vi "Serialize To Inputs.vi"(0 "Input 6":variant, 4 "Input 5":variant, 6 "Input 4":variant, 8 "Input 3":variant, 9 "Input 2":variant, 10 "Input 1":variant, 11 "Base Queue in":refnum<class "Base Queue.lvclass">) -> (3 "Base Queue out":refnum<class "Base Queue.lvclass">)   [LabVIEW 2021, in "jettl.lvlib" / "Base Queue.lvlib" / "Base Queue.lvclass"]
uses:
  Base Queue.lvclass
  Base Queue.lvclass/Base Queue.ctl
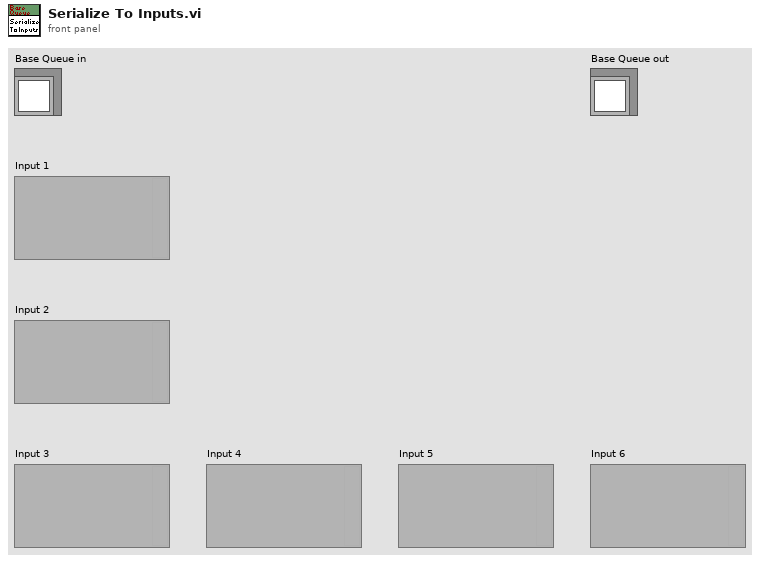
[diagram p1: front panel]
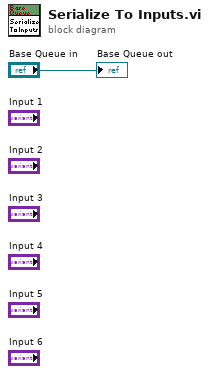
[diagram p0: block diagram]
diagram:
  "Base Queue out" <- "Base Queue in"
